vi "901.vi"(6 "error in (no error)":errorcluster, 7 "Cluster":T1, 8 "String":string, 9 "Array":dbl[](array[numeric]), 10 "Boolean":bool, 11 "Numeric":dbl) -> (0 "String 2":string, 1 "Array 2":dbl[](array[numeric]), 2 "Boolean 2":bool, 3 "Numeric 2":dbl, 4 "error in (no error) 2":errorcluster, 5 "Cluster 2":T1)   [LabVIEW 2009]
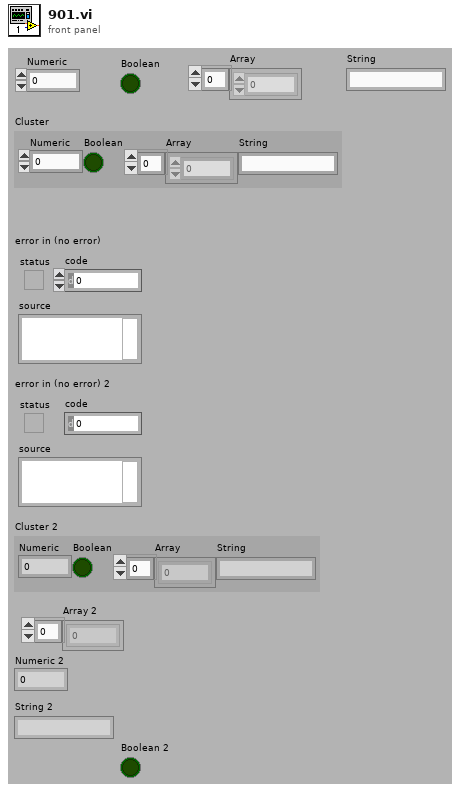
[diagram p1: front panel]
types:
  T1 = cluster{"Numeric":dbl, "Boolean":bool, "Array":dbl[], "String":string}
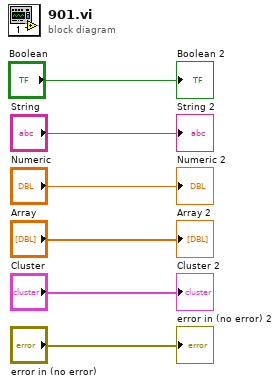
[diagram p0: block diagram]
diagram:
  "Boolean 2" <- "Boolean"
  "error in (no error) 2" <- "error in (no error)"
  "Cluster 2" <- "Cluster"
  "Array 2" <- "Array"
  "Numeric 2" <- "Numeric"
  "String 2" <- "String"
